vi "PV ActiveLine - DisplayControlScreensave.vi"(7 "W/R":bool, 8 "Fehler (Eingang)":errorcluster, 9 "screensave control in":u16(ring) items=["off", "10 min", "30 min", "1 h", "2 h", "8 h"], 11 "Referenz in":refnum<visa-resource-name>) -> (0 "Cluster (Ausgang)":errorcluster, 1 "screensave control out":i8(ring) items=["off", "10 min", "30 min", "1 h", "2 h", "8 h"], 3 "Referenz out":refnum<visa-resource-name>)   [LabVIEW 2013, in "PV ActiveLine.lvlib"]
doc: "DCS - Display Control Screensave\n\nTransmit: DCS [,a]\nReceive: a\n\nScreensave,\na =\n0 –> Off (default)\n1 –> After 10 minutes\n2 –> After 30 minutes\n3 –> After 1 hour\n4 –> After 2 hours\n5 –> After 8 hours"
uses:
  <instrlib>/PV ActiveLine/PV ActiveLine.lvlib
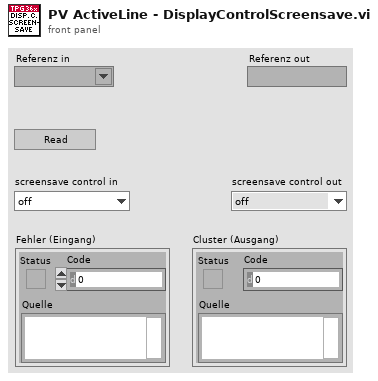
[diagram p1: front panel]
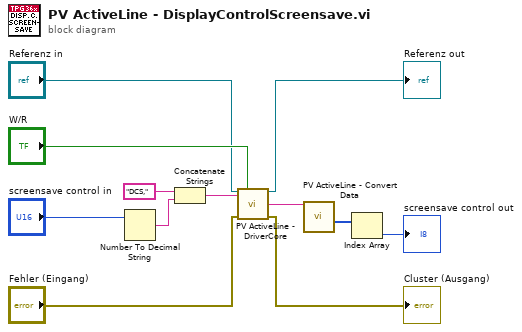
[diagram p0: block diagram]
diagram:
  n1 = Number To Decimal String(number="screensave control in") -> (decimal integer string=w8:string)  [unwired: 1 in]
  n2 = Concatenate Strings("DCS,", w8) -> (w10:string)
  n3 = call <instrlib>:"PV ActiveLine - DriverCore.vi"("Referenz in"="Referenz in", "Write/Read"="W/R", "Command"=w10, "Fehler (Eingang)"="Fehler (Eingang)") -> ("Referenz out"=→"Referenz out":refnum<visa-resource-name>, "String Out"=w3:string, "Cluster (Ausgang)"=→"Cluster (Ausgang)":errorcluster)  [unwired: 9 in]
  n4 = call <instrlib>:"PV ActiveLine - Convert Data.vi"("String in"=w3) -> ("Integer Out"=w2:i32[])  [unwired: 7 in, 3 out]
  n5 = Index Array(array=w2) -> (element=→"screensave control out":i32)  [unwired: 1 in]
